vi "Count up U16.vi"(9 "reset":bool=TRUE, 10 "increment":bool=TRUE) -> (2 "count out":u16)   [LabVIEW 2020]
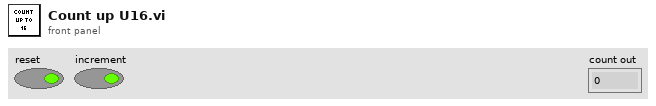
[diagram p1: front panel]
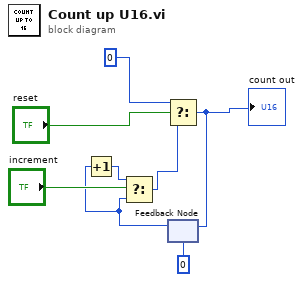
[diagram p0: block diagram]
diagram:
  n1 = feedback #1(u16 0) -> (w1:u16)
  n2 = Increment(x=w1) -> (x+1=w2:u16)
  n3 = Select(t=w2, s="increment", f=w1) -> (s? t:f=w5:u16)
  n4 = Select(t=u16 0, s="reset", f=w5) -> (s? t:f=w4:u16)
  "count out" <- w4
  n5 = feedback-in #1(w4) -> ()
